vi "To Origin File.vi"(4 "Y":dbl[](array[numeric]), 8 "X":dbl[](array[numeric]), 11 "Prefix":string) -> (3 "Text":string)   [LabVIEW 2018]
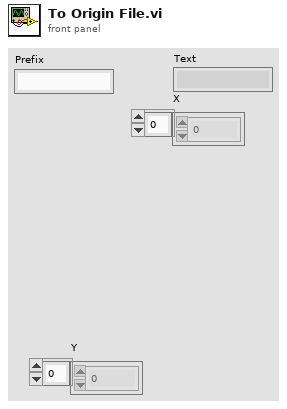
[diagram p1: front panel]
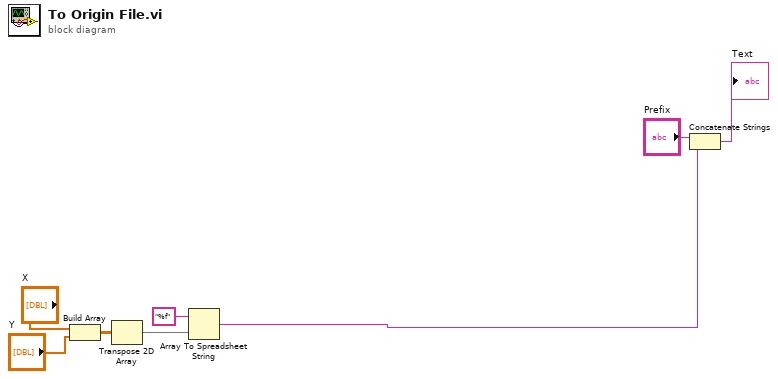
[diagram p0: block diagram]
diagram:
  n1 = Build Array("X", "Y") -> (w6:dbl[][])
  n2 = Transpose 2D Array(2D array=w6) -> (transposed array=w7:dbl[][])
  n3 = Array To Spreadsheet String(array=w7, 3:"%f" ("format string")) -> (spreadsheet string=w2:string)  [unwired: 1 in]
  n4 = Concatenate Strings("Prefix", w2) -> (→"Text":string)
